vi "niRFUtil RFHS FIFO Create Error Cluster.vi"(7 "error in (no error)":errorcluster, 9 "fifo return value":i32) -> (8 "error  out":errorcluster, 10 "is error?":bool)   [LabVIEW 2015, in "niRFUtil.lvlib"]
uses:
  niRFUtil.lvlib
  niRFUtil RFHS FIFO Error Codes.ctl
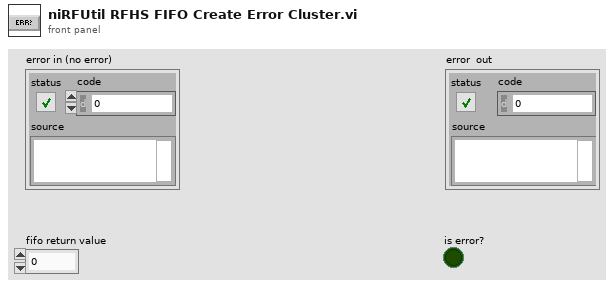
[diagram p1: front panel]
types:
  T1 = typedef "niRFUtil.lvlib/niRFUtil RFHS FIFO Error Codes.ctl" = i32
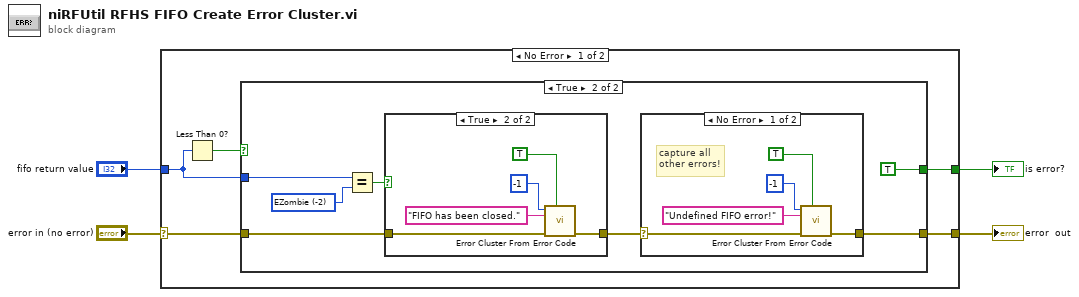
[diagram p0: block diagram]
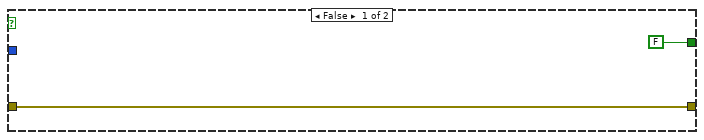
[diagram p2: hidden frame]
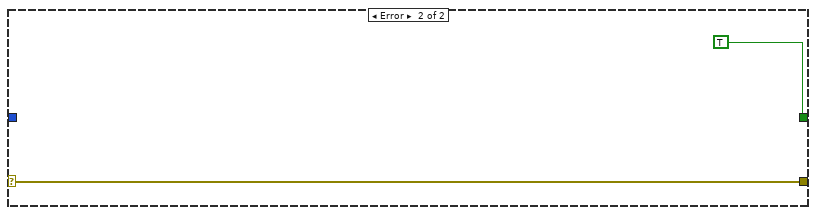
[diagram p5: hidden frame]
diagram:
  n1 = case shown="No Error" "error in (no error)" {
    selector: "error in (no error)" -> [w8 w32]
    tunnel: [w6 w32] -> w3
    tunnel: "fifo return value" -> [w7 _]
    tunnel: [w5 TRUE] -> w1
    frame No Error {
      n2 = Less Than 0?(x=w7) -> (x < 0?=w9:bool)
      n3 = case shown="True" w9 {
        tunnel: w8 -> [w11 w15]
        tunnel: w7 -> [_ w17]
        tunnel: [w11 w13] -> w6
        tunnel: [FALSE TRUE] -> w5
        frame False {
        }
        frame True {
          w16 = T1 -2 items=["OK"=1, "EAgain"=-1, "EZombie"=-2] ("Fifo error states")
          n4 = Equal?(x=w17, y=w16) -> (x = y?=w18:bool)
          n5 = case shown="True" w18 {
            tunnel: w15 -> [w25 w30]
            tunnel: [w25 w29] -> w14
            frame False {
            }
            frame True {
              n6 = call <vilib>:"Error Cluster From Error Code.vi"("show call chain? (False)"=TRUE, "error in (no error)"=w30, "error message (\"\")"="FIFO has been closed." ("error message (\"\")"), "error code (0)"=-1) -> ("error out"=w29:errorcluster)  [unwired: 5 in]
            }
          }
          n7 = case shown="No Error" w14 {
            selector: w14 -> [w20 w24]
            tunnel: [w19 w24] -> w13
            frame No Error {
              # "capture all\nother errors!"
              n8 = call <vilib>:"Error Cluster From Error Code.vi"("show call chain? (False)"=TRUE, "error in (no error)"=w20, "error message (\"\")"="Undefined FIFO error!" ("error message (\"\")"), "error code (0)"=-1) -> ("error out"=w19:errorcluster)  [unwired: 5 in]
            }
            frame Error {
              # "No need to capture error, because\nwe have an error cluster already"
            }
          }
        }
      }
    }
    frame Error {
    }
  }
  "error  out" <- w3
  "is error?" <- w1
